vi "testGetTagContent--Subroutine.vi"(8 "error in (no error)":errorcluster, 11 "TestCase in":refnum<class "EasyXMLTest.lvclass">) -> (0 "error out":errorcluster, 3 "TestCase out":refnum<class "EasyXMLTest.lvclass">)   [LabVIEW 2013, in "EasyXMLTest.lvclass"]
doc: "Verify that error in is not overwritten"
uses:
  EasyXMLTest.lvclass
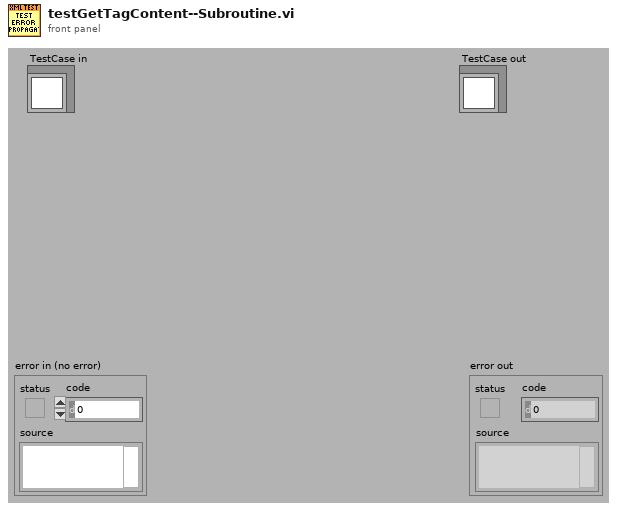
[diagram p1: front panel]
types:
  T1 = enum32{"invalid priority", "background priority", "normal priority", "above normal priority", "high priority", "time critical priority", "subroutine"}
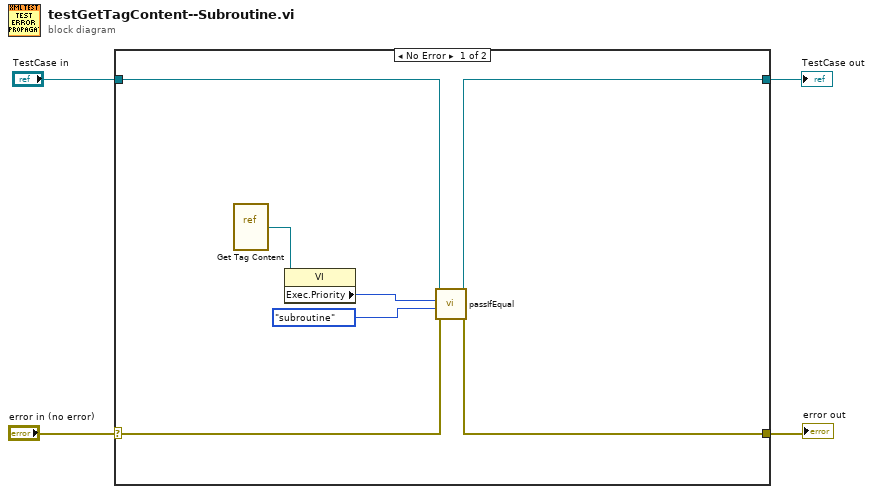
[diagram p0: block diagram]
diagram:
  n1 = case shown="No Error" "error in (no error)" {
    selector: "error in (no error)" -> [w6 w13]
    tunnel: [w5 w13] -> w3
    tunnel: [w7 w12] -> w1
    tunnel: "TestCase in" -> [w8 w12]
    frame No Error {
      n2 = vi-ref "Get Tag Content.vi"() -> (w11:refnum<vi>)
      n3 = property class="VI"(reference=w11) -> ("Exec.Priority"=w10:T1)  [unwired: 1 in, 2 out]
      n4 = call-dynamic "passIfEqual.vi"("error in (no error)"=w6, "y"=T1."subroutine" ("Execution:Priority"), "x"=w10, "TestCase in"=w8) -> ("error out"=w5:errorcluster, "TestCase out"=w7:refnum<class "EasyXMLTest.lvclass">)  [unwired: 6 in]
    }
    frame Error {
    }
  }
  "error out" <- w3
  "TestCase out" <- w1
